vi "Content Rect Bounds Separator.vi"(8 "error in (no error)":errorcluster, 10 "Boolean":bool, 11 "ListBx in":refnum<class "ListBox.lvclass">) -> (0 "error out":errorcluster, 3 "ListBx out":refnum<class "ListBox.lvclass">)   [LabVIEW 2015, in "ListBox.lvclass"]
uses:
  ListBox.lvclass
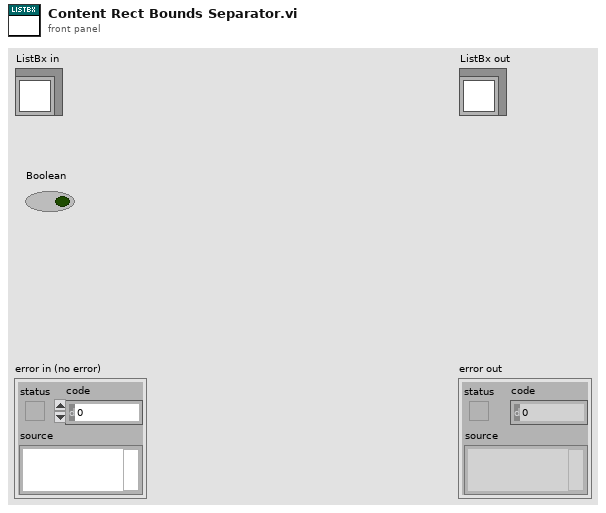
[diagram p1: front panel]
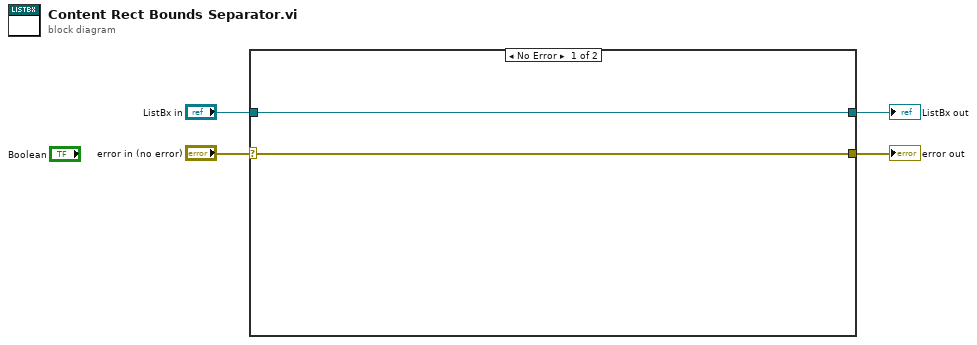
[diagram p0: block diagram]
diagram:
  n1 = case shown="No Error" "error in (no error)" {
    selector: "error in (no error)" -> [w5 w8]
    tunnel: [w5 w8] -> w3
    tunnel: [w6 w7] -> w1
    tunnel: "ListBx in" -> [w6 w7]
    frame No Error {
    }
    frame Error {
    }
  }
  "error out" <- w3
  "ListBx out" <- w1
